vi "Follow Aircraft on Mini Map.vi"(8 "Error In":errorcluster, 11 "Aircraft ID":u8) -> (0 "error out":errorcluster)   [LabVIEW 2014]
uses:
  Aircraft Information/Sub VI/Get Aircraft GPS.vi
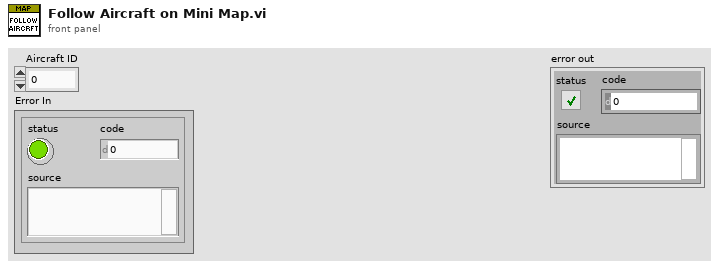
[diagram p1: front panel]
types:
  T1 = typedef "Aircraft GPS Data.ctl" = cluster{"Latitude (degrees)":dbl, "Longitude (degrees)":dbl, "Altitude (m)":dbl, "Fix Type":T2, "HDOP (cm)":u16, "VDOP (cm)":u16, "Ground Speed (m/s)":dbl, "Coarse Over Ground (degrees)":u16, "Number of Satellites":u8}
  T2 = typedef "GPS Fix Type.ctl" = enum16{"No Fix 0", "No Fix 1", "2D Fix", "3D Fix", "DGPS", "RTK"}
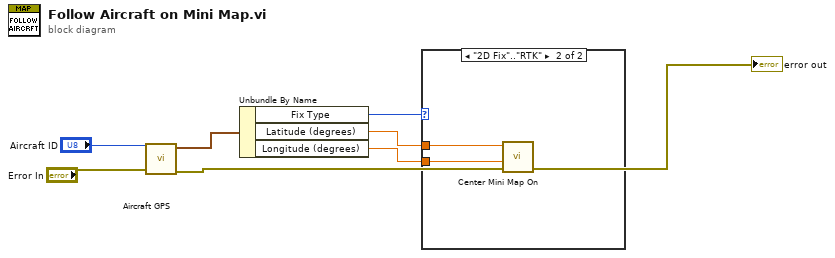
[diagram p0: block diagram]
diagram:
  n1 = call-poly "Aircraft GPS.vi"("Error In"="Error In", "Aircraft ID"="Aircraft ID") -> ("Error Out"=→"error out":errorcluster, "Aircraft GPS Data Out"=w4:T1)  [unwired: 8 in]
  n2 = Unbundle By Name(w4) -> ("Fix Type"=w1:T2, "Latitude (degrees)"=w3:dbl, "Longitude (degrees)"=w2:dbl)
  n3 = case shown="\"2D Fix\"..\"RTK\"" w1 {
    tunnel: w3 -> [_ w9]
    tunnel: w2 -> [_ w8]
    frame "No Fix 0", Default {
    }
    frame "2D Fix".."RTK" {
      n4 = call "Center Mini Map On.vi"("lng"=w8, "lat"=w9) -> ()  [unwired: 9 in, 1 out]
    }
  }
